vi "Read Data Test.vi"(8 "error in (no error)":errorcluster caption="entrée d'erreur (pas d'erreur)", 11 "Database Altyor en entrée":refnum<class "Database Altyor Packaging.lvclass">) -> (0 "error out":errorcluster caption="sortie d'erreur", 3 "Database Altyor en sortie":refnum<class "Database Altyor Packaging.lvclass">)   [LabVIEW 2020, in "Library Instrument & Equipement.lvlib" / "Library Database.lvlib" / "Database Altyor Packaging.lvclass"]
uses:
  Database Altyor Packaging.lvclass
  C:/Users/ngarcin/OneDrive - Altyor/Standard TB/Class/Database/Database drivers/Database Drivers.lvclass
  <vilib>/addons/database/_DB Variant To Data/Database Variant To Data.xnode
  Database Altyor Packaging.lvclass/Database Altyor Packaging.ctl
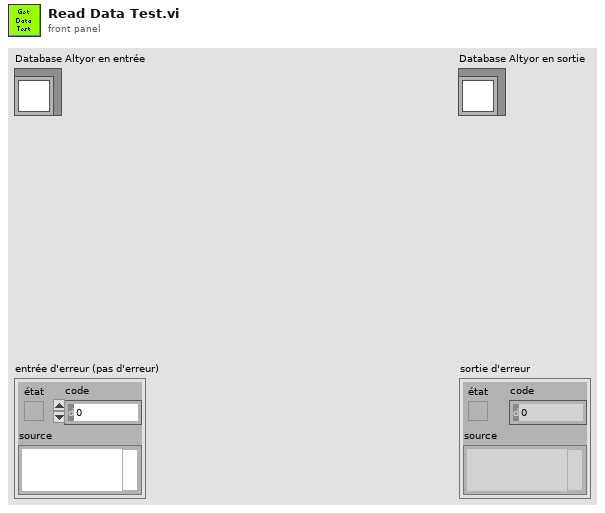
[diagram p1: front panel]
types:
  T1 = cluster{"Key_Test":u32, "idPackaging":u32, "Name":string, "Name":string, "SerialNumber":string}[]
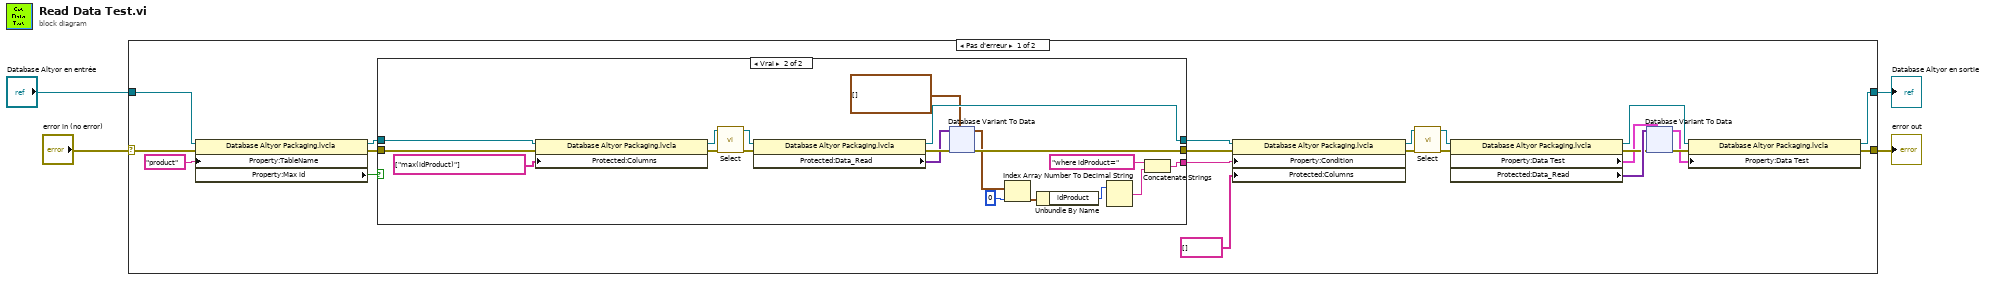
[diagram p0: block diagram]
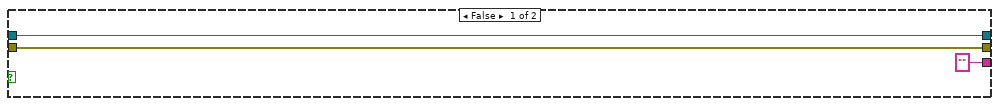
[diagram p2: hidden frame]
diagram:
  n1 = case shown="Pas d'erreur" "error in (no error)" {
    selector: "error in (no error)" -> [w24 w256]
    tunnel: [w21 w256] -> w3
    tunnel: [w19 w255] -> w1
    tunnel: "Database Altyor en entrée" -> [w23 w255]
    frame No Error {
      n2 = property class="Database Altyor Packaging.lvcla"(reference=w23, error in=w24, "Property:TableName"="product" ("TableName")) -> (reference out=w12:refnum<class "Database Altyor Packaging.lvclass">, error out=w11:errorcluster, "Property:Max id"=w13:bool)
      n3 = case shown="Vrai" w13 {
        tunnel: [w27 w42] -> w10
        tunnel: [w28 w44] -> w8
        tunnel: ["" w35] -> w6
        tunnel: w12 -> [w28 w33]
        tunnel: w11 -> [w27 w32]
        frame False {
        }
        frame True {
          n4 = property class="Database Altyor Packaging.lvcla"(reference=w33, error in=w32, "Protected:Columns"=string[] ["max(idProduct)"] ("Columns")) -> (reference out=w47:refnum<class "Database Altyor Packaging.lvclass">, error out=w48:errorcluster)
          n5 = call-dynamic "Select.vi"("error in (no error)"=w48, "Database Drivers en entrée"=w47) -> ("error out"=w46:errorcluster, "Database Drivers en sortie"=w45:refnum<class "Database Altyor Packaging.lvclass">)  [unwired: 8 in]
          n6 = property class="Database Altyor Packaging.lvcla"(reference=w45, error in=w46) -> (reference out=w44:refnum<class "Database Altyor Packaging.lvclass">, error out=w43:errorcluster, "Protected:Data_Read"=w41:variant[][])
          n7 = xnode "Database Variant To Data"("database variant"=w41, "error in (no error)"=w43, "type"=cluster{"idProduct":u32}[] [] ("Main Data")) -> ("data"=w40:cluster{"idProduct":u32}[], "error out"=w42:errorcluster)
          n8 = Index Array(array=w40, index=0 ("indice")) -> (element=w31:cluster{"idProduct":u32})
          n9 = Unbundle By Name(w31) -> ("idProduct"=w37:u32)
          n10 = Number To Decimal String(number=w37) -> (decimal integer string=w36:string)  [unwired: 1 in]
          n11 = Concatenate Strings("where idProduct=" ("chaîne"), w36) -> (w35:string)
        }
      }
      n12 = property class="Database Altyor Packaging.lvcla"(reference=w8, error in=w10, "Property:Condition"=w6, "Protected:Columns"=string[] [] ("Columns")) -> (reference out=w7:refnum<class "Database Altyor Packaging.lvclass">, error out=w9:errorcluster)
      n13 = call-dynamic "Select.vi"("error in (no error)"=w9, "Database Drivers en entrée"=w7) -> ("error out"=w25:errorcluster, "Database Drivers en sortie"=w26:refnum<class "Database Altyor Packaging.lvclass">)  [unwired: 8 in]
      n14 = property class="Database Altyor Packaging.lvcla"(reference=w26, error in=w25) -> (reference out=w20:refnum<class "Database Altyor Packaging.lvclass">, error out=w17:errorcluster, "Property:Data Test"=w15:T1, "Protected:Data_Read"=w18:variant[][])
      n15 = xnode "Database Variant To Data"("database variant"=w18, "error in (no error)"=w17, "type"=w15) -> ("data"=w14:T1, "error out"=w16:errorcluster)
      n16 = property class="Database Altyor Packaging.lvcla"(reference=w20, error in=w16, "Property:Data Test"=w14) -> (reference out=w19:refnum<class "Database Altyor Packaging.lvclass">, error out=w21:errorcluster)
    }
    frame Error {
    }
  }
  "error out" <- w3
  "Database Altyor en sortie" <- w1
